vi "initialise.vi"(8 "error in (no error)":errorcluster, 11 "GenericPlugin in":refnum<class "StimulatorAK101022TCP.lvclass">) -> (0 "error out":errorcluster, 3 "GenericPlugin out":refnum<class "StimulatorAK101022TCP.lvclass">)   [LabVIEW 2010, in "StimulatorAK101022TCP.lvclass"]
doc: "The dynamic dispatch-version of this VI initalises the plug-in object by allocating and initalising any dynamic resources need."
uses:
  StimulatorAK101022TCP.lvclass
  StimulatorDL090503Scaffold/StimulatorDL090503Scaffold/StimulatorDL090503Scaffold.lvclass
  StimulatorAK101022TCP.lvclass/StimulatorAK101022TCP.ctl
  StringGenerator/GenericStringGenerator/GenericStringGenerator/GenericStringGenerator.lvclass
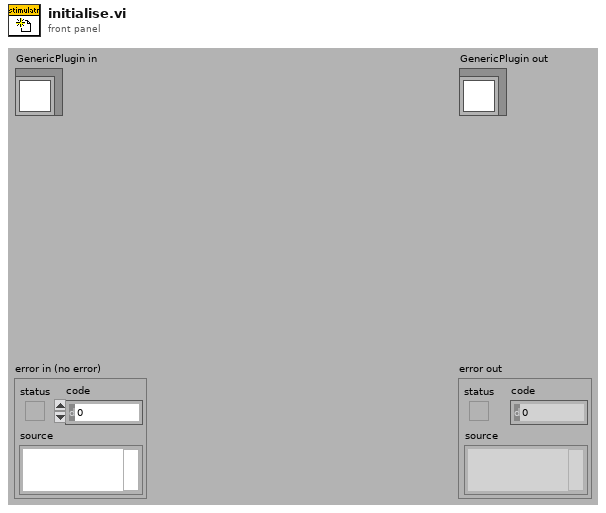
[diagram p1: front panel]
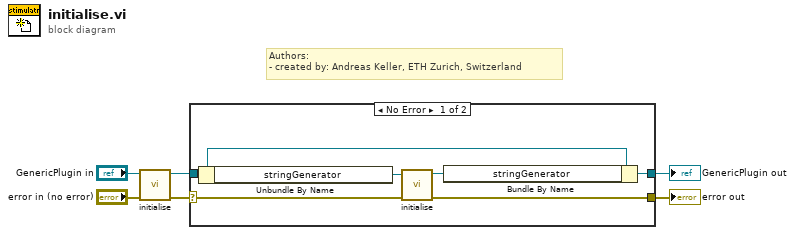
[diagram p0: block diagram]
diagram:
  # "Authors: \n- created by: Andreas Keller, ETH Zurich, Switzerland"
  n1 = call-parent "initialise.vi"("error in (no error)"="error in (no error)", "GenericPlugin in"="GenericPlugin in") -> ("error out"=w4:errorcluster, "GenericPlugin out"=w2:refnum<class "StimulatorAK101022TCP.lvclass">)  [unwired: 8 in]
  n2 = case shown="No Error" w4 {
    selector: w4 -> [w12 w14]
    tunnel: [w11 w14] -> w3
    tunnel: [w9 w13] -> w1
    tunnel: w2 -> [w10 w13]
    frame No Error {
      n3 = Unbundle By Name(w10) -> ("stringGenerator"=w7:refnum<class "GenericStringGenerator.lvclass">)
      n4 = call-dynamic "initialise.vi"("error in (no error)"=w12, "GenericPlugin in"=w7) -> ("error out"=w11:errorcluster, "GenericPlugin out"=w8:refnum<class "GenericStringGenerator.lvclass">)  [unwired: 8 in]
      n5 = Bundle By Name(cluster=w10, "stringGenerator"=w8) -> (w9:refnum<class "StimulatorAK101022TCP.lvclass">)
    }
    frame Error {
    }
  }
  "error out" <- w3
  "GenericPlugin out" <- w1
